vi "Read Report error and stop.vi"(8 "error in (no error)":errorcluster, 11 "Da Base in":refnum<class "Template Module.lvclass">) -> (0 "error out":errorcluster, 2 "Report error and stop":bool, 3 "Da Base out":refnum<class "Template Module.lvclass">)   [LabVIEW 2019, in "Template Module.lvclass"]
uses:
  Template Module.lvclass
  Template Module.lvclass/Template Module.ctl
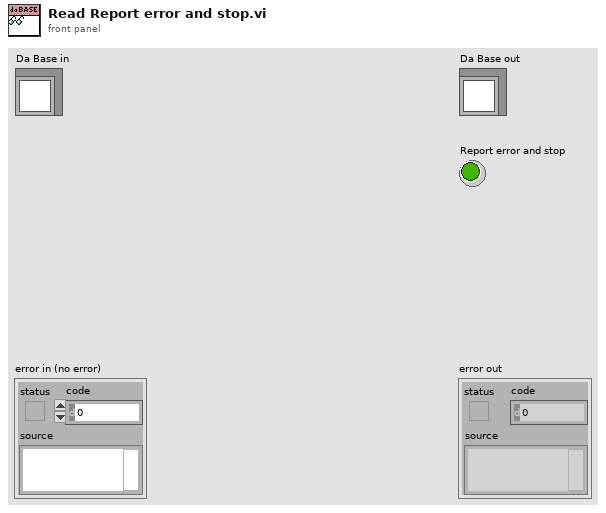
[diagram p1: front panel]
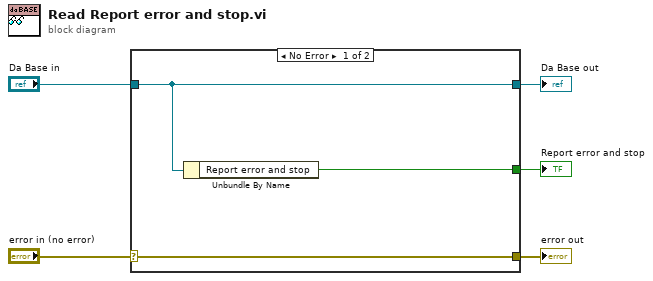
[diagram p0: block diagram]
diagram:
  n1 = case shown="No Error" "error in (no error)" {
    selector: "error in (no error)" -> [w8 w9]
    tunnel: [w8 w9] -> w4
    tunnel: [w7 w10] -> w2
    tunnel: "Da Base in" -> [w7 w10]
    tunnel: [w6 _] -> w1
    frame No Error {
      n2 = Unbundle By Name(w7) -> ("Report error and stop"=w6:bool)
    }
    frame Error {
    }
  }
  "error out" <- w4
  "Da Base out" <- w2
  "Report error and stop" <- w1
